vi "worksheet write boolean.vi"(6 "format":u32, 7 "value":i32, 8 "error in (no error)":errorcluster, 9 "col":u16, 10 "row":u32, 11 "worksheet":u32) -> (0 "error out":errorcluster, 3 "function return":u32(ring))   [LabVIEW 8.6]
doc: "lxw_error worksheet_write_boolean(lxw_worksheet worksheet, lxw_row_t row, lxw_col_t col, int value, lxw_format format);"
uses:
  pending_lvxlsxwriter/xlsxwriter.dll
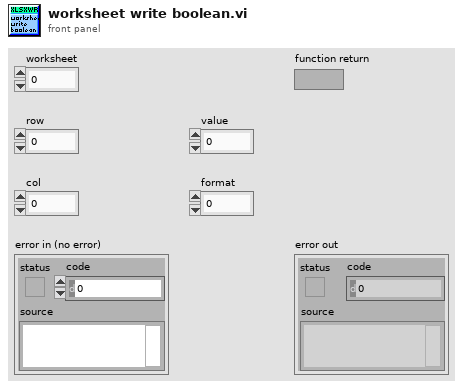
[diagram p1: front panel]
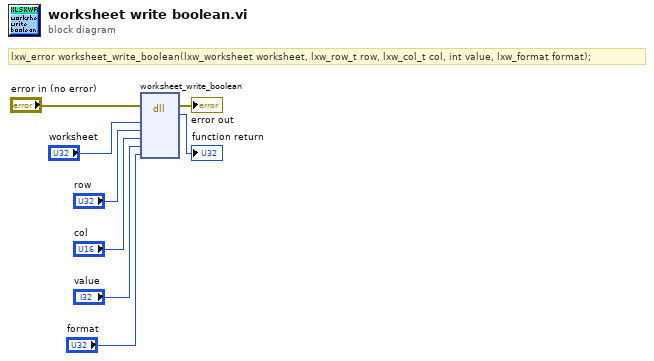
[diagram p0: block diagram]
diagram:
  # "lxw_error worksheet_write_boolean(lxw_worksheet worksheet, lxw_row_t row, lxw_col_t col, int value, lxw_format format);"
  n1 = dll-call lib="C:/Users/WDAGUtilityAccount/Desktop/pending_lvxlsxwriter/xlsxwriter.*" fn="worksheet_write_boolean"(error in="error in (no error)", "worksheet"="worksheet", "row"="row", "col"="col", "value"="value", "format"="format") -> (error out=→"error out":errorcluster, →"function return":u32)  [unwired: 7 in, 1 out]
